vi "弹窗-提示-刷新失败.vi"() -> ()   [LabVIEW 2017]
panel:
  in  "确定":bool
  # "本次导出已取消"
  # "数据导出过程中刷新数据失败"
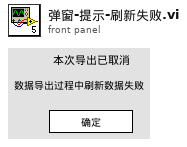
[diagram p1: front panel]
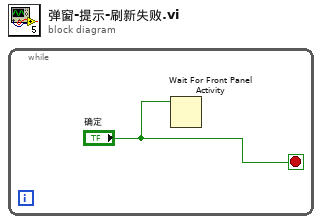
[diagram p0: block diagram]
diagram:
  n1 = while {
    stop <- "确定" stop-if-true
    n2 = Wait For Front Panel Activity(3:"确定") -> ()  [unwired: 2 in, 1 out]
  }
